vi "Draw Pov.vi"(10 "pov":i32=45, 11 "Draw Area Size":T1) -> (3 "2D Picture":picture)   [LabVIEW 2021]
uses:
  <vilib>/Utility/miscctls.llb/LVBoundsTypeDef.ctl
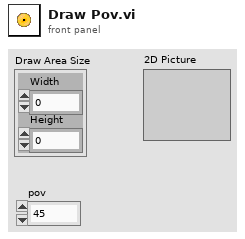
[diagram p1: front panel]
types:
  T1 = typedef "LVBoundsTypeDef.ctl" = cluster{"Width":u32, "Height":u32}
  T2 = cluster{"Width":u16, "Style":enum32{"Solid", "Dash", "Dot", "DashDot", "DashDotDot"}}
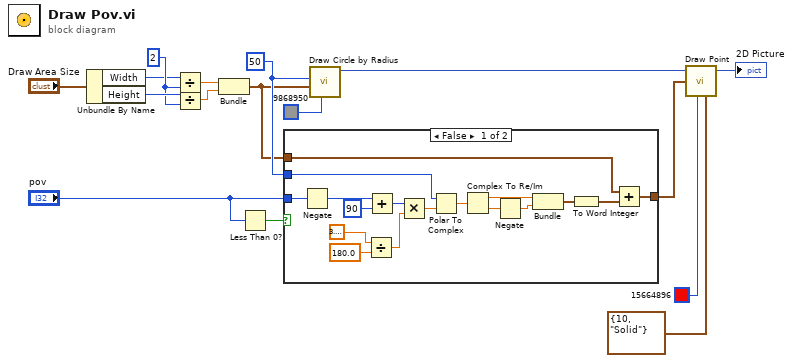
[diagram p0: block diagram]
diagram:
  w15 = u32 2 ("y")
  w5 = i16 50 ("radius")
  n1 = Unbundle By Name("Draw Area Size") -> ("Width"=w12:u32, "Height"=w16:u32)
  n2 = Divide(x=w12, y=w15) -> (x/y=w14:dbl)
  n3 = Divide(x=w16, y=w15) -> (x/y=w13:dbl)
  n4 = Bundle(w14, w13) -> (w2:cluster{dbl, dbl})  [unwired: 1 in]
  n5 = Less Than 0?(x="pov") -> (x < 0?=w6:bool)
  n6 = case shown="False" w6 {
    tunnel: w5 -> [w25 _]
    tunnel: "pov" -> [w20 _]
    tunnel: w2 -> [w24 w34]
    tunnel: [w23 w34] -> w3
    frame False {
      n7 = Negate(x=w20) -> (-x=w19:i32)
      n8 = Divide(x=3.141592653589793, y=180.0) -> (x/y=w31:dbl)
      n9 = Add(x=w19, y=90) -> (x+y=w17:i32)
      n10 = Multiply(x=w17, y=w31) -> (x*y=w32:dbl)
      n11 = Polar To Complex(1:w32, 2:w25) -> (0:w26:cdb)
      n12 = Complex To Re/Im(x + iy=w26) -> (x=w22:dbl, y=w28:dbl)
      n13 = Negate(x=w28) -> (-x=w21:dbl)
      n14 = Bundle(w22, w21) -> (w27:cluster{dbl, dbl})  [unwired: 1 out]
      n15 = To Word Integer(number=w27) -> (16bit integer=w33:cluster{i16, i16})
      n16 = Add(x=w24, y=w33) -> (x+y=w23:cluster{dbl, dbl})
    }
    frame True {
    }
  }
  n17 = call <vilib>:"Draw Circle by Radius.vi"("color(black)"=u32 9868950, "pixel center"=w2, "radius"=w5) -> ("new picture"=w9:picture)  [unwired: 8 in]
  n18 = call <vilib>:"Draw Point.vi"("picture"=w9, "point(x,y)"=w3, "color(black)"=u32 15664896, "pen"=T2 {"Width"=10, "Style"=enum."Solid"}) -> ("new picture"=→"2D Picture":picture)  [unwired: 5 in]
